vi "get Active Device.vi"(11 "IO in":refnum<class "IO.lvclass">) -> (3 "Active Device":T1=enum."None")   [LabVIEW 2021, in "IO.lvclass"]
uses:
  IO.lvclass
  Memory Map/Active Device.ctl
  IO.lvclass/IO.ctl
  Memory Map/Memory Map.lvclass/Memory Map.ctl
  Memory Map/Memory Map.lvclass
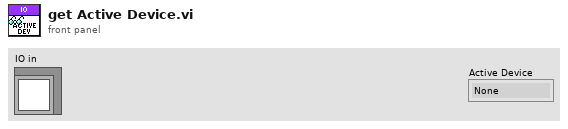
[diagram p1: front panel]
types:
  T1 = typedef "Memory Map.lvclass/Active Device.ctl" = enum16{"Error", "None", "RAM", "EEPROM", "VIA"}
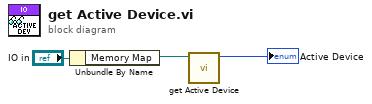
[diagram p0: block diagram]
diagram:
  n1 = Unbundle By Name("IO in") -> ("Memory Map"=w2:refnum<class "Memory Map.lvclass">)
  n2 = call "get Active Device.vi"("Memory Map in"=w2) -> ("Active Device"=→"Active Device":T1)  [unwired: 10 in]
